vi "niFpgaPID_PDCore.vi"(0 "setpoint":sgl, 1 "reset? (F)":bool, 3 "channel (0)":u8, 5 "process variable":sgl, 7 "manual control":T3, 12 "gains":T2 {"filter coefficient" min=0 max=1; "proportional gain" step=0.125}, 13 "output range":T5={"output high (Inf)"=inf, "output low (-Inf)"=-inf}, 14 "setpoint weighting":T4={"proportional weighting (1)"=1.0, "derivative weighting (0)"=0.0} {"derivative weighting (0)" min=0 max=1; "proportional weighting (1)" min=0 max=1}) -> (4 "output":sgl, 6 "error":sgl, 8 "actions":T1)   [LabVIEW 2020]
uses:
  <vilib>/rvi/Analysis/control/PID/Typedef/niFpgaPID_OutputRange.ctl
  <vilib>/rvi/Analysis/control/PID/Typedef/niFpgaPID_SetpointWeightings.ctl
  <vilib>/rvi/Analysis/control/PID/Typedef/niFpgaPID_ManualControl.ctl
  <vilib>/rvi/Analysis/control/PID/Typedef/niFpgaPID_PDGains.ctl
  <vilib>/rvi/Analysis/control/PID/Typedef/niFpgaPID_PDActions.ctl
  <vilib>/rvi/Analysis/control/PID/Typedef/niFpgaPID_PDErrors.ctl
  <vilib>/rvi/Analysis/control/PID/Typedef/niFpgaPID_PDParameters.ctl
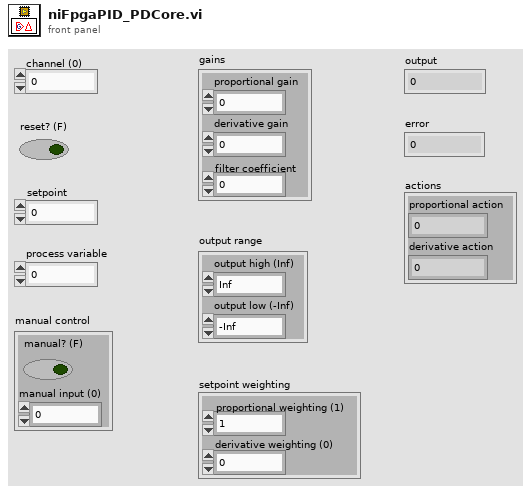
[diagram p1: front panel]
types:
  T1 = typedef "niFpgaPID_PDActions.ctl" = cluster{"proportional action":sgl, "derivative action":sgl}
  T2 = typedef "niFpgaPID_PDGains.ctl" = cluster{"proportional gain":sgl, "derivative gain":sgl, "filter coefficient":sgl}
  T3 = typedef "niFpgaPID_ManualControl.ctl" = cluster{"manual? (F)":bool, "manual input (0)":sgl}
  T4 = typedef "niFpgaPID_SetpointWeightings.ctl" = cluster{"proportional weighting (1)":sgl, "derivative weighting (0)":sgl}
  T5 = typedef "niFpgaPID_OutputRange.ctl" = cluster{"output high (Inf)":sgl, "output low (-Inf)":sgl}
  T6 = typedef "niFpgaPID_PDParameters.ctl" = cluster{"Kp":sgl, "Kd":sgl, "manual?":bool, "beta":sgl}
  T7 = typedef "niFpgaPID_PDErrors.ctl" = cluster{"error with beta":sgl, "error with gamma":sgl}
  T8 = typedef "niFpgaPID_PDState.ctl" = cluster{"e(k-1) with gamma":sgl, "output (k-1)":sgl, "uD(k-1)":sgl}
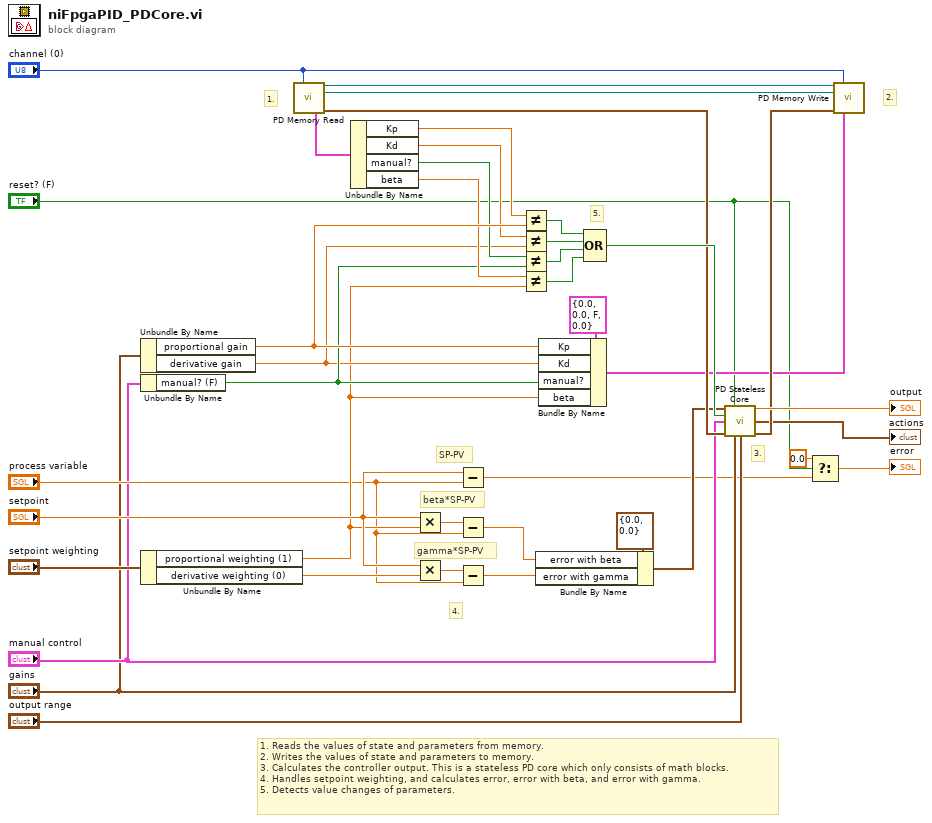
[diagram p0: block diagram]
diagram:
  # "1. Reads the values of state and parameters from memory.\n2. Writes the values of state and parameters to memory.\n3. Calculates the controller output. This is a stateless PD core which only consists of math blocks.\n4. Handles setpoint weighting, and calculates error, error with beta, and error with gamma.\n5. Detects value changes of parameters."
  # "SP-PV"
  # "beta*SP-PV"
  # "gamma*SP-PV"
  # "5."
  # "4."
  # "3."
  # "2."
  # "1."
  n1 = Unbundle By Name("gains") -> ("proportional gain"=w36:sgl, "derivative gain"=w28:sgl)
  n2 = Unbundle By Name("manual control") -> ("manual? (F)"=w29:bool)
  n3 = Unbundle By Name("setpoint weighting") -> ("proportional weighting (1)"=w21:sgl, "derivative weighting (0)"=w38:sgl)
  n4 = call "PD Memory Read"("channel (0)"="channel (0)") -> ("data memory out"=w16:refnum<k21>, "manual memory out"=w15:refnum<k21>, "parameters out"=w19:T6, "state out"=w34:T8)  [unwired: 11 in]
  n5 = Unbundle By Name(w19) -> ("Kp"=w33:sgl, "Kd"=w32:sgl, "manual?"=w31:bool, "beta"=w30:sgl)
  n6 = Multiply(x="setpoint", y=w21) -> (x*y=w1:sgl)
  n7 = Multiply(x="setpoint", y=w38) -> (x*y=w2:sgl)
  n8 = Subtract(x="setpoint", y="process variable") -> (x-y=w6:sgl)
  n9 = Subtract(x=w1, y="process variable") -> (x-y=w18:sgl)
  n10 = Subtract(x=w2, y="process variable") -> (x-y=w17:sgl)
  n11 = Not Equal?(x=w33, y=w36) -> (x != y?=w10:bool)
  n12 = Not Equal?(x=w32, y=w28) -> (x != y?=w27:bool)
  n13 = Not Equal?(x=w31, y=w29) -> (x != y?=w26:bool)
  n14 = Not Equal?(x=w30, y=w21) -> (x != y?=w25:bool)
  n15 = Bundle By Name(cluster=T7 {"error with beta"=0.0, "error with gamma"=0.0} ("errors"), "error with beta"=w18, "error with gamma"=w17) -> (w13:T7)
  n16 = Bundle By Name(cluster=T6 {"Kp"=0.0, "Kd"=0.0, "manual?"=FALSE, "beta"=0.0} ("parameters"), "Kp"=w36, "Kd"=w28, "manual?"=w29, "beta"=w21) -> (w8:T6)
  n17 = Compound Arithmetic op=OR(w10, w27, w26, w25) -> (w37:bool)
  n18 = call "PD Stateless Core"("errors"=w13, "reset? (F)"="reset? (F)", "enable bumpless transfer? (F)"=w37, "manual control"="manual control", "state in"=w34, "gains"="gains", "output range"="output range") -> ("output"=→"output":sgl, "actions"=→"actions":T1, "state out"=w35:T8)  [unwired: 6 in]
  n19 = Select(t=sgl 0.0, s="reset? (F)", f=w6) -> (s? t:f=→"error":sgl)
  n20 = call "PD Memory Write"("data memory in"=w16, "channel (0)"="channel (0)", "manual memory in"=w15, "state in"=w35, "parameters in"=w8) -> ()  [unwired: 11 in]
